vi "Add Trigger Channel.vi"(8 "error in":errorcluster, 10 "name":string, 11 "acyclic frames section":T1 format="%.0x") -> (0 "error out":errorcluster, 3 "acyclic frame trigger":T1 format="%.0x")   [LabVIEW 2020, in "Ballard MIL-STD-1553 Scripting.lvlib"]
uses:
  Ballard MIL-STD-1553 Scripting.lvlib
  <vilib>/NI VeriStand/Custom Device API/Custom Device Item Ref.ctl
  <vilib>/NI VeriStand/Custom Device API/Custom Device Channel.ctl
  <vilib>/NI VeriStand/Custom Device API/Custom Device Channel Type.ctl
  Constants.vi
  <vilib>/NI VeriStand/Custom Device API/Custom Device API.lvlib
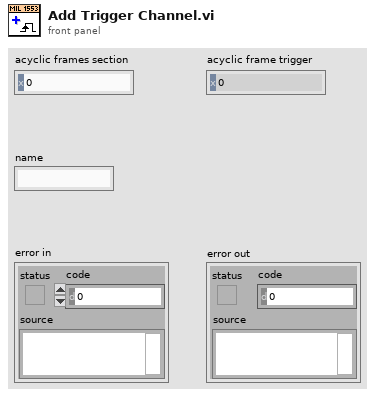
[diagram p1: front panel]
types:
  T1 = typedef "Custom Device API.lvlib/Custom Device Item Ref.ctl" = u64
  T2 = typedef "Custom Device API.lvlib/Custom Device Channel.ctl" = cluster{"Type":T3, "Units":string, "Default Value":dbl, "Faultable":bool, "Scalable":bool}
  T3 = typedef "Custom Device API.lvlib/Custom Device Channel Type.ctl" = enum16{"Input", "Output"}
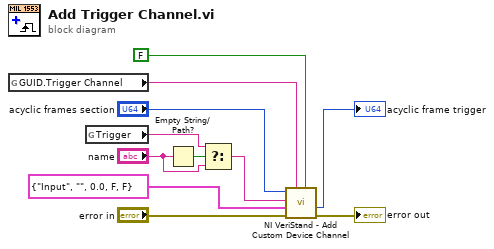
[diagram p0: block diagram]
diagram:
  n1 = global read "Constants.vi" "GUID.Trigger Channel"() -> (w1:string)
  n2 = global read "Constants.vi" "Trigger"() -> (w3:string)
  n3 = Empty String/Path?(string/path="name") -> (empty?=w5:bool)
  n4 = Select(t=w3, s=w5, f="name") -> (s? t:f=w2:string)
  n5 = call <vilib>:"NI VeriStand - Add Custom Device Channel.vi"("Highlight? (F)"=FALSE, "GUID (Default Channel)"=w1, "error in (no error)"="error in", "Channel"=T2 {"Type"=enum."Input", "Units"="", "Default Value"=0.0, "Faultable"=FALSE, "Scalable"=FALSE}, "Channel Name"=w2, "Parent Ref in"="acyclic frames section") -> ("error out"=→"error out":errorcluster, "Channel Ref"=→"acyclic frame trigger":T1)  [unwired: 2 in, 2 out]
